vi "Write DATA.vi"(8 "error in (no error)":errorcluster, 10 "DATA":T1, 11 "Queue in":refnum<class "Queue.lvclass">) -> (0 "error out":errorcluster, 3 "Queue out":refnum<class "Queue.lvclass">)   [LabVIEW 2020, in "Data Communication Transmitter.lvlib" / "Queue.lvclass"]
uses:
  Classes/Children/Intra-Application/Children/With Data/Children/Queues/Queue.lvclass
  Classes/Children/Intra-Application/Children/With Data/Children/Queues/Queue.lvclass/Queue.ctl
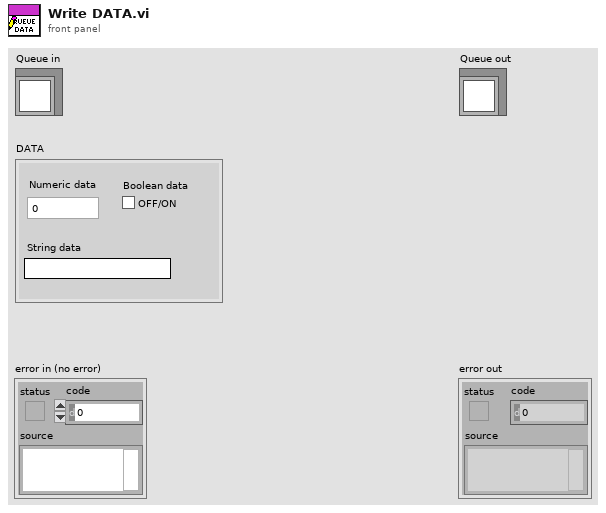
[diagram p1: front panel]
types:
  T1 = cluster{"Numeric data":dbl, "String data":string, "Boolean data":bool}
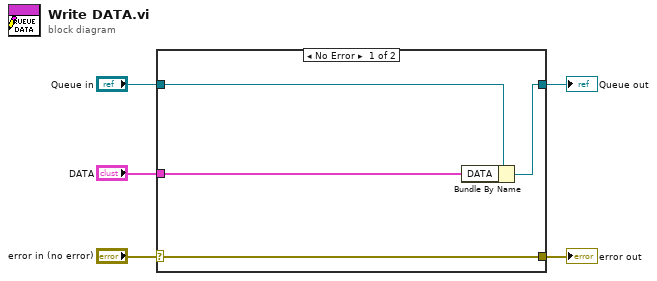
[diagram p0: block diagram]
diagram:
  n1 = case shown="No Error" "error in (no error)" {
    selector: "error in (no error)" -> [w9 w10]
    tunnel: [w9 w10] -> w4
    tunnel: [w7 w11] -> w2
    tunnel: "Queue in" -> [w8 w11]
    tunnel: "DATA" -> [w6 _]
    frame No Error {
      n2 = Bundle By Name(cluster=w8, "DATA"=w6) -> (w7:refnum<class "Queue.lvclass">)
    }
    frame Error {
    }
  }
  "error out" <- w4
  "Queue out" <- w2
